vi "Configure Trigger Impedance.vi"(8 "error in (no error)":errorcluster, 10 "impedence (50 Ohm)":enum16{"50 Ohm", "1 kOhm"}(ring), 11 "VISA resource name":refnum<visa-resource-name>) -> (0 "error out":errorcluster, 3 "VISA resource name out":refnum<visa-resource-name>)   [LabVIEW 2019, in "Pulse Rider PG-1000.lvlib"]
doc: "This command sets the trigger input impedance; it can be 50 Ohm or 1KOhm\n\nImpedance: trigger input impedance '50ohm', '1kohm'"
uses:
  <instrlib>/LV_PulseRiderPG1000/Pulse Rider PG-1000.lvlib
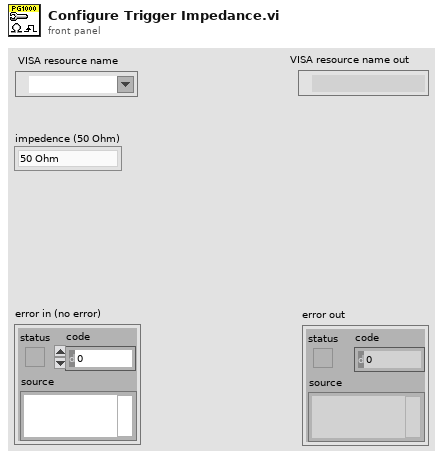
[diagram p1: front panel]
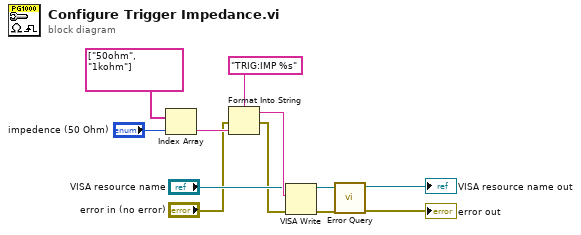
[diagram p0: block diagram]
diagram:
  n1 = Index Array(array=string[] ["50ohm", "1kohm"], index="impedence (50 Ohm)") -> (element=w5:string)
  n2 = Format Into String(format string="TRIG:IMP %s", error in="error in (no error)", w5) -> (resulting string=w9:string, error out=w1:errorcluster)  [unwired: 1 in]
  n3 = VISA Write(VISA resource name="VISA resource name", write buffer=w9, error in (no error)=w1) -> (VISA resource name out=w12:refnum<visa-resource-name>, error out=w11:errorcluster)  [unwired: 1 out]
  n4 = call <instrlib>:"Error Query.vi"("error in (no error)"=w11, "VISA resource name"=w12) -> ("error out"=→"error out":errorcluster, "VISA resource name out"=→"VISA resource name out":refnum<visa-resource-name>)  [unwired: 6 in, 2 out]
